vi "IntakeCODE.vi"(9 "Intake Button B":bool, 11 "Intake Button A":bool) -> (2 "Intake Value":string)   [LabVIEW 2018]
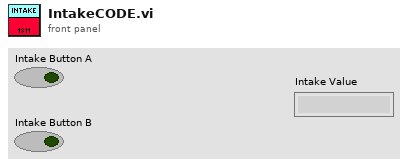
[diagram p1: front panel]
types:
  T1 = typedef "WPI_SwitchDevRef.ctl" = cluster{"DevStatus":errorcluster, "DIO Channel":T2, "CntIndex":T3, "Normally Closed":bool}
  T2 = typedef "FPGA_DIOChannel.ctl" = enum8{"DIO 0", "DIO 1", "DIO 2", "DIO 3", "DIO 4", "DIO 5", "DIO 6", "DIO 7", "DIO 8", "DIO 9", "DIO MXP 0", "DIO MXP 1", "DIO MXP 2", "DIO MXP 3", "DIO MXP 4", "DIO MXP 5", "DIO MXP 6", "DIO MXP 7", "DIO MXP 8", "DIO MXP 9", "DIO MXP 10", "DIO MXP 11", "DIO MXP 12", "DIO MXP 13", "DIO MXP 14", "DIO MXP 15", "SPI Port CS1", "SPI Port CS2", "SPI Port CS3", "SPI Port MISO", "SPI Port MOSI", "Invalid"}
  T3 = typedef "FPGA_CounterCtrSystemIndex.ctl" = enum8{"Ctr 0", "Ctr 1", "Ctr 2", "Ctr 3", "Ctr 4", "Ctr 5", "Ctr 6", "Ctr 7", "Invalid"}
  T4 = typedef "WPI_MotorControlDeviceRef.ctl" = cluster{"DeviceStatus":errorcluster, "Type":T5, "PWM":cluster{"PWM Channel":T6, "DeadBand":T7}, "CAN":cluster{"Device Number":u8, "SetOutput VI Ref":variant, "GetOutput VI Ref":variant, "Enable VI Ref":variant, "Disable VI Ref":variant, "Data":variant}, "Invert":bool, "DIO PWM":cluster{"PWM \"Enable\" Channel":T6, "DIOChannel":T2, "PWM Rate":dbl}}
  T5 = typedef "WPI_MotorControlType.ctl" = enum16{"PWM", "CAN", "DIO PWM"}
  T6 = typedef "FPGA_DIOPWMChannel.ctl" = enum8{"PWM 0", "PWM 1", "PWM 2", "PWM 3", "PWM 4", "PWM 5", "PWM 6", "PWM 7", "PWM 8", "PWM 9", "PWM MXP 0", "PWM MXP 1", "PWM MXP 2", "PWM MXP 3", "PWM MXP 4", "PWM MXP 5", "PWM MXP 6", "PWM MXP 7", "PWM MXP 8", "PWM MXP 9", "Invalid"}
  T7 = typedef "WPI_PWMDeadband.ctl" = cluster{"Name":string, "maxPositivePwm":i32, "minPositivePwm":i32, "centerPwm":i32, "maxNegativePwm":i32, "minNegativePwm":i32, "angularRange":u16}
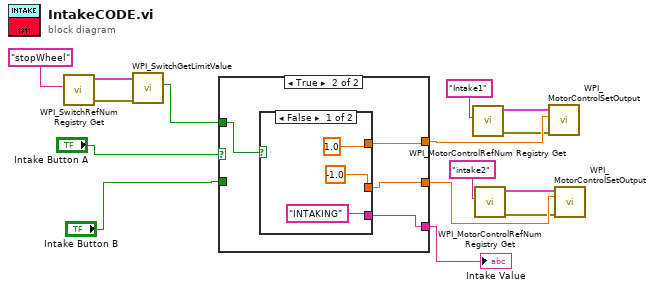
[diagram p0: block diagram]
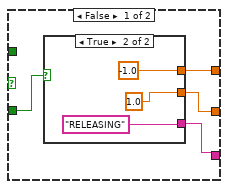
[diagram p2: hidden frame]
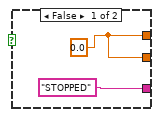
[diagram p3: hidden frame]
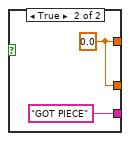
[diagram p4: hidden frame]
diagram:
  n1 = call <vilib>:"WPI_SwitchRefNum Registry Get.vi"("refnum name"="stopWheel") -> ("error out"=w5:errorcluster, "SwitchDevRef"=w4:T1)  [unwired: 9 in]
  n2 = call <vilib>:"WPI_SwitchGetLimitValue.vi"("error in (no error)"=w5, "SwitchDevRef"=w4) -> ("Switch Pressed"=w2:bool)  [unwired: 7 in, 2 out]
  n3 = case shown="True" "Intake Button A" {
    tunnel: [w18 w25] -> w13
    tunnel: [w19 w26] -> w12
    tunnel: "Intake Button B" -> [w17 _]
    tunnel: [w16 w28] -> w1
    tunnel: w2 -> [_ w27]
    frame False {
      n4 = case shown="True" w17 {
        tunnel: [w21 -1.0 ("Output")] -> w19
        tunnel: [w21 1.0 ("Output")] -> w18
        tunnel: ["STOPPED" ("Intake Value") "RELEASING" ("refnum name")] -> w16
        frame False {
          w21 = 0.0 ("Output")
        }
        frame True {
        }
      }
    }
    frame True {
      n5 = case shown="False" w27 {
        tunnel: ["INTAKING" ("refnum name") "GOT PIECE" ("refnum name")] -> w28
        tunnel: [1.0 ("Output") w32] -> w26
        tunnel: [-1.0 ("Output") w32] -> w25
        frame False {
        }
        frame True {
          w32 = 0.0 ("Output")
        }
      }
    }
  }
  "Intake Value" <- w1
  n6 = call <vilib>:"WPI_MotorControlRefNum Registry Get.vi"("refnum name"="Intake1") -> ("error out"=w10:errorcluster, "MotorControlDevRef"=w11:T4)  [unwired: 9 in]
  n7 = call <vilib>:"WPI_MotorControlRefNum Registry Get.vi"("refnum name"="intake2") -> ("error out"=w8:errorcluster, "MotorControlDevRef"=w9:T4)  [unwired: 9 in]
  n8 = call <vilib>:"WPI_MotorControlSetOutput.vi"("error in (no error)"=w10, "Output"=w12, "MotorControlDevRef"=w11) -> ()  [unwired: 6 in, 3 out]
  n9 = call <vilib>:"WPI_MotorControlSetOutput.vi"("error in (no error)"=w8, "Output"=w13, "MotorControlDevRef"=w9) -> ()  [unwired: 6 in, 3 out]
